vi "Clean Up Children.vi"(8 "error in (no error)":errorcluster, 9 "Folder Names":refnum<class "UTF-8 String.lvclass">[](array[class]), 10 "Parent Tag":refnum<class "UTF-8 String.lvclass">, 11 "Tree In":refnum<vi>) -> (0 "error out":errorcluster, 1 "Folder Names Dup":refnum<class "UTF-8 String.lvclass">[](array[class]), 2 "Parent Tag Dup":refnum<class "UTF-8 String.lvclass">, 3 "Tree Out":refnum<vi>)   [LabVIEW 2020, in "Tree Browser.lvlib"]
doc: "Deletes any children immediately under a parent node which don't exist on disk."
uses:
  Tree Browser.lvlib
  Types/UTF-8 String/UTF-8 String.lvclass
  Types/UTF-8 String/UTF-8 String.lvclass/UTF-8 String.ctl
  cc51fbc4-9572-46a5-8299-7a6ed0f38a74.vi
  Private/Conversion/Text as String.vi
  Private/Conversion/Polymorphic VIs/Text as String (UTF-8 String).vi
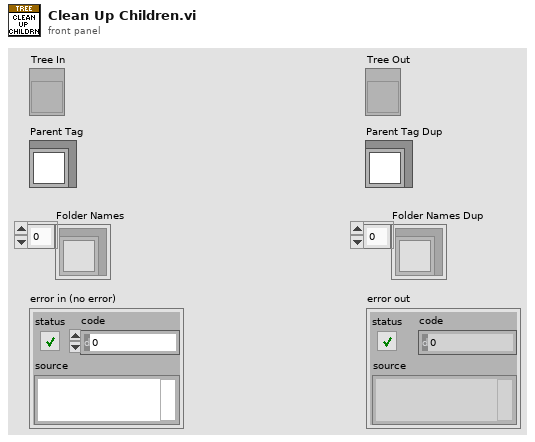
[diagram p1: front panel]
types:
  T1 = typedef "G-Unicode.lvlib/Encoded UTF-8 String.ctl" = string
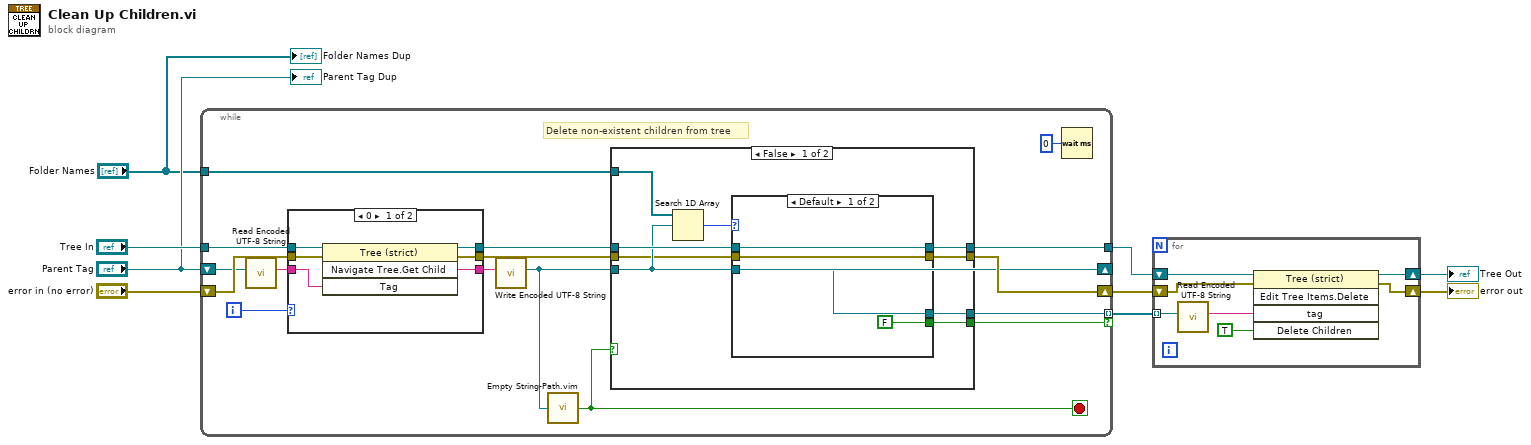
[diagram p0: block diagram]
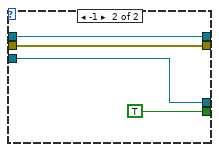
[diagram p2: hidden frame]
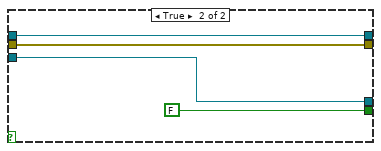
[diagram p3: hidden frame]
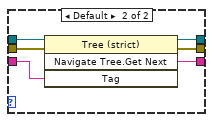
[diagram p4: hidden frame]
diagram:
  n1 = while {
    tunnel: "Tree In" -> [w25]
    shift-right: [w10] -> _
    shift-left: "Parent Tag" -> [w13]
    tunnel: "Folder Names" -> [w21]
    tunnel: [w20] -> w4
    shift-right: [w17] -> w2
    shift-left: "error in (no error)" -> [w19]
    tunnel: [w16] -> w5 mode=indexing if=w15
    i -> [w24]
    stop <- w23 stop-if-true
    # "Delete non-existent children from tree"
    n2 = call "Read Encoded UTF-8 String.vi"("UTF-8 String"=w13) -> ("Encoded UTF-8 String"=w12:T1)  [unwired: 10 in]
    n3 = case shown="0" w24 {
      tunnel: w25 -> [w52 w58]
      tunnel: w12 -> [w51 w53]
      tunnel: [w50 w57] -> w11
      tunnel: [w49 w56] -> w22
      tunnel: w19 -> [w48 w55]
      tunnel: [w47 w54] -> w18
      frame 0 {
        n4 = invoke class="Tree (strict)" method="Navigate Tree.Get Child"(reference=w52, error in=w48, "Tag"=w51) -> (reference out=w49:refnum<vi>, error out=w47:errorcluster, "Navigate Tree:Get Child"=w50:string)  [unwired: 1 in, 1 out]
      }
      frame Default {
        n5 = invoke class="Tree (strict)" method="Navigate Tree.Get Next"(reference=w58, error in=w55, "Tag"=w53) -> (reference out=w56:refnum<vi>, error out=w54:errorcluster, "Navigate Tree:Get Next Item"=w57:string)  [unwired: 1 in, 1 out]
      }
    }
    n6 = call "Write Encoded UTF-8 String.vi"("Encoded UTF-8 String"=w11) -> ("UTF-8 String"=w10:refnum<class "UTF-8 String.lvclass">)  [unwired: 10 in]
    n7 = call "Empty String-Path.vim"("String/Path"=w10) -> ("Empty?"=w23:bool)
    n8 = case shown="False" w23 {
      tunnel: w22 -> [w33 w46]
      tunnel: w21 -> [w32 _]
      tunnel: w10 -> [w31 w44]
      tunnel: [w30 w46] -> w20
      tunnel: w18 -> [w29 w45]
      tunnel: [w28 w45] -> w17
      tunnel: [w27 w44] -> w16
      tunnel: [w26 FALSE] -> w15
      frame False {
        n9 = Search 1D Array(1D array=w32, element=w31) -> (index of element=w34:i32)  [unwired: 1 in]
        n10 = case shown="Default" w34 {
          tunnel: w33 -> [w38 w41]
          tunnel: w31 -> [w36 w42]
          tunnel: [w38 w41] -> w30
          tunnel: w29 -> [w37 w40]
          tunnel: [w37 w40] -> w28
          tunnel: [w36 w42] -> w27
          tunnel: [FALSE TRUE] -> w26
          frame Default {
          }
          frame -1 {
          }
        }
      }
      frame True {
      }
    }
    n11 = Wait (ms)(milliseconds to wait=u32 0) -> ()  [unwired: 1 out]
  }
  n12 = for {
    tunnel: w5 -> [w64] mode=indexing
    shift-right: [w60] -> w1
    shift-left: w2 -> [w61]
    shift-right: [w62] -> w3
    shift-left: w4 -> [w63]
    n13 = call "Read Encoded UTF-8 String.vi"("UTF-8 String"=w64) -> ("Encoded UTF-8 String"=w59:T1)  [unwired: 10 in]
    n14 = invoke class="Tree (strict)" method="Edit Tree Items.Delete"(reference=w63, error in=w61, "tag"=w59, "Delete Children"=TRUE ("Delete Children?")) -> (reference out=w62:refnum<vi>, error out=w60:errorcluster)  [unwired: 1 in, 3 out]
  }
  "Tree Out" <- w3
  "error out" <- w1
  "Parent Tag Dup" <- "Parent Tag"
  "Folder Names Dup" <- "Folder Names"
